vi "tsapp_configure_can_regs.vi"(10 "簇":T1, 11 "路径输入":path) -> (2 "返回类型":i32, 3 "路径输出":path)   [LabVIEW 2019]
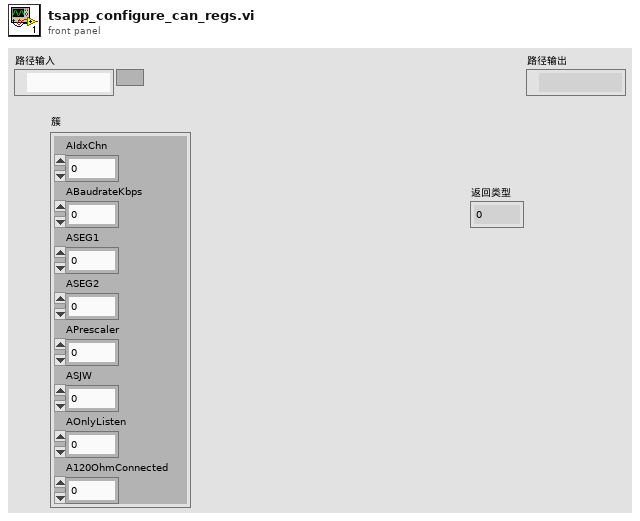
[diagram p1: front panel]
types:
  T1 = cluster{"AIdxChn":i32, "ABaudrateKbps":sgl, "ASEG1":i32, "ASEG2":i32, "APrescaler":i32, "ASJW":i32, "AOnlyListen":i32, "A120OhmConnected":i32}
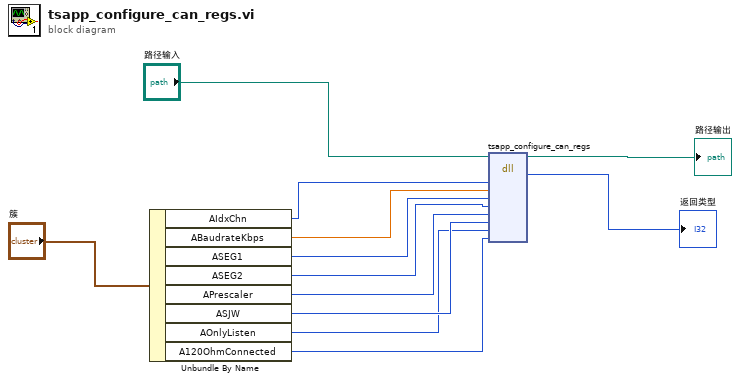
[diagram p0: block diagram]
diagram:
  n1 = Unbundle By Name("簇") -> ("AIdxChn"=w9:i32, "ABaudrateKbps"=w8:sgl, "ASEG1"=w6:i32, "ASEG2"=w7:i32, "APrescaler"=w5:i32, "ASJW"=w4:i32, "AOnlyListen"=w1:i32, "A120OhmConnected"=w2:i32)
  n2 = dll-call lib="C:/Users/XYY/Desktop/LabView Demo/TSCAN_LB2018_V1.3_20220301/Config/TSMaster.dll" fn="tsapp_configure_can_regs"(path in="路径输入", "AIdxChn"=w9, "ABaudrateKbps"=w8, "ASEG1"=w6, "ASEG2"=w7, "APrescaler"=w5, "ASJW"=w4, "AOnlyListen"=w1, "A120OhmConnected"=w2) -> (path out=→"路径输出":path, "返回类型"=→"返回类型":i32)  [unwired: 10 in, 1 out]
